vi "test Log Span Size.vi"(8 "error in":errorcluster, 11 "TestCase in":refnum<class "Embedded Data Logger System Tests.lvclass">) -> (0 "error out":errorcluster, 3 "TestCase out":refnum<class "Embedded Data Logger System Tests.lvclass">)   [LabVIEW 2018, in "Embedded Data Logger System Tests.lvclass"]
uses:
  Embedded Data Logger System Tests.lvclass
  <vilib>/addons/_JKI Toolkits/VI Tester/TestCase.llb/TestCase.lvclass
  C:/Program Files (x86)/National Instruments/LabVIEW 2018/vi.lib/addons/_JKI Toolkits/VI Tester/TestCase.llb/TestCase.lvclass
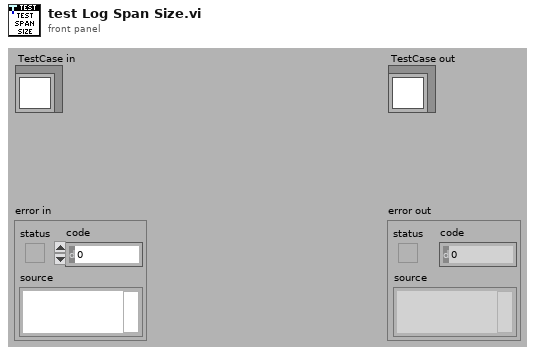
[diagram p1: front panel]
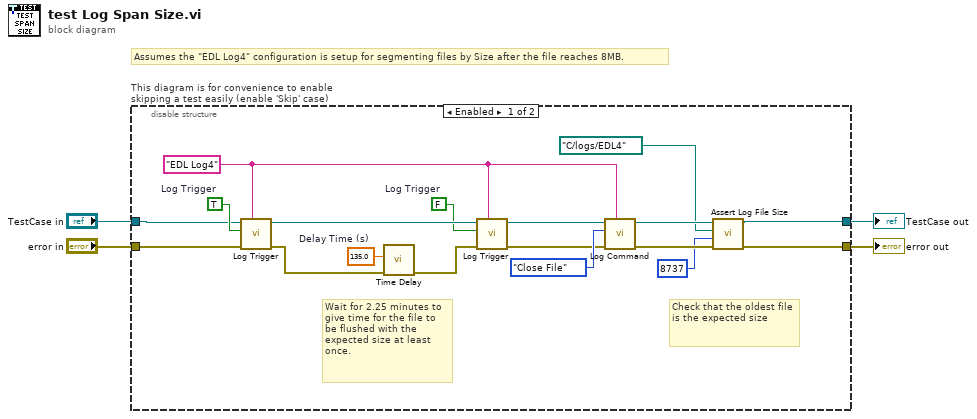
[diagram p0: block diagram]
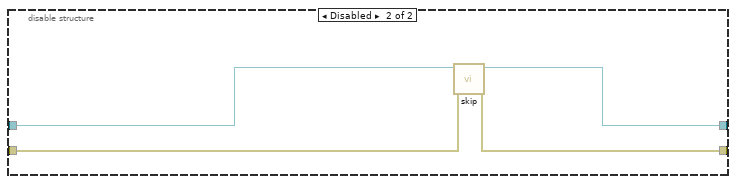
[diagram p2: hidden frame]
diagram:
  # "Assumes the \"EDL Log4\" configuration is setup for segmenting files by Size after the file reaches 8MB."
  n1 = disable-structure "This diagram is for convenience to enable skipping a test easily (enable 'Skip' case)" shown="Enabled" {
    disable-tunnel: "TestCase in" -> [w15 w26]
    disable-tunnel: [w9 w24] -> w1
    disable-tunnel: [w7 w25] -> w3
    disable-tunnel: "error in" -> [w16 w23]
    frame Enabled {
      w11 = "EDL Log4" ("Embedded Data Logger File Name")
      w19 = FALSE  # Log Trigger
      w17 = 135.0  # Delay Time (s)
      w18 = TRUE  # Log Trigger
      # "Check that the oldest file is the expected size"
      # "Wait for 2.25 minutes to give time for the file to be flushed with the expected size at least once."
      n2 = call "Log Trigger.vi"("Embedded Data Logger File Name"=w11, "error in"=w16, "Log Trigger"=w18, "Embedded Data Logger System Tests in"=w15) -> ("error out"=w21:errorcluster, "Embedded Data Logger System Tests out"=w20:refnum<class "Embedded Data Logger System Tests.lvclass">)  [unwired: 6 in]
      n3 = call "Time Delay"("error in (no error)"=w21, "Delay Time (s)"=w17) -> ("error out"=w22:errorcluster)  [unwired: 9 in]
      n4 = call "Log Trigger.vi"("Embedded Data Logger File Name"=w11, "error in"=w22, "Log Trigger"=w19, "Embedded Data Logger System Tests in"=w20) -> ("error out"=w13:errorcluster, "Embedded Data Logger System Tests out"=w12:refnum<class "Embedded Data Logger System Tests.lvclass">)  [unwired: 6 in]
      n5 = call "Log Command.vi"("Embedded Data Logger File Name"=w11, "error in"=w13, "Log Command"=enum16{"Idle", "Open File", "Close File"}."Close File", "Embedded Data Logger System Tests in"=w12) -> ("error out"=w8:errorcluster, "Embedded Data Logger System Tests out"=w10:refnum<class "Embedded Data Logger System Tests.lvclass">)  [unwired: 6 in]
      n6 = call "Assert Log File Size.vi"("error in"=w8, "Expected size of file in bytes"=i64 8737, "file path"=path "C:/logs/EDL4", "Embedded Data Logger System Tests in"=w10) -> ("error out"=w7:errorcluster, "Embedded Data Logger System Tests out"=w9:refnum<class "Embedded Data Logger System Tests.lvclass">)  [unwired: 6 in]
    }
    frame Disabled {
      # "skip test result while test is under development"
      n7 = call <vilib>:"skip.vi"("error in (no error)"=w23, "TestCase in"=w26) -> ("error out"=w25:errorcluster, "TestCase out"=w24:refnum<class "Embedded Data Logger System Tests.lvclass">)  [unwired: 8 in]
    }
  }
  "error out" <- w3
  "TestCase out" <- w1
